vi "Get Item BG Color.vi"(0 "Tree Reference In":refnum<vi>, 1 "Tag (Current)":string, 5 "error in (no error)":errorcluster, 9 "Column # (0)":i32) -> (14 "Tree Reference Out":refnum<vi>, 15 "Duplicate Tag":string, 19 "error out":errorcluster)   [LabVIEW 2015, in "QuickVIew.lvlib"]
doc: "Gets cell BG colorTLB Prime - Application Template 1.3.0.24\nNorm Kirchner, NI Systems Engineering - NI\nCopyright (c) 2014, NI"
uses:
  QuickVIew.lvlib
panel:
  out "Cell BG Color":u32(colorbox)
  # "VI INPUTS"
  # "VI OUTPUTS"
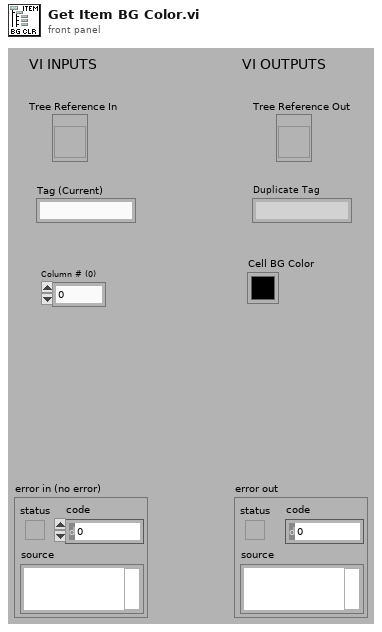
[diagram p1: front panel]
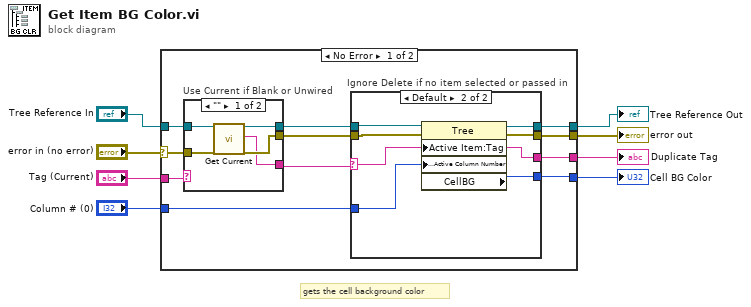
[diagram p0: block diagram]
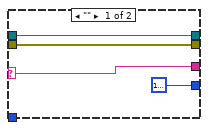
[diagram p2: hidden frame]
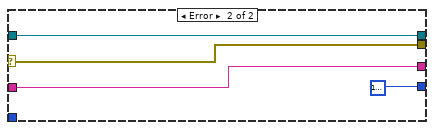
[diagram p4: hidden frame]
diagram:
  # "gets the cell background color"
  n1 = case shown="No Error" "error in (no error)" {
    selector: "error in (no error)" -> [w17 w41]
    tunnel: "Tree Reference In" -> [w19 w42]
    tunnel: [w16 w42] -> w7
    tunnel: [w15 w41] -> w6
    tunnel: "Tag (Current)" -> [w18 w40]
    tunnel: "Column # (0)" -> [w11 _]
    tunnel: [w10 w40] -> w2
    tunnel: [w9 u32 16777226 ("Cell BG Color")] -> w1
    frame No Error {
      n2 = case "Use Current if Blank or Unwired" shown="\"\"" w18 {
        selector: w18 -> [_ w36]
        tunnel: [w34 w38] -> w14
        tunnel: w19 -> [w35 w38]
        tunnel: [w33 w37] -> w13
        tunnel: w17 -> [w32 w37]
        tunnel: [w31 w36] -> w12
        frame "" {
          n3 = call "Get Current.vi"("Tree Reference In"=w35, "error in (no error)"=w32) -> ("Tree Reference Out"=w34:refnum<vi>, "Current Tag"=w31:string, "error out"=w33:errorcluster)  [unwired: 14 in, 1 out]
        }
        frame Default {
        }
      }
      n4 = case "Ignore Delete if no item selected or passed in" shown="Default" w12 {
        selector: w12 -> [w21 w25]
        tunnel: [w23 w27] -> w16
        tunnel: [w22 w26] -> w15
        tunnel: w14 -> [w23 w30]
        tunnel: w13 -> [w22 w29]
        tunnel: w11 -> [_ w28]
        tunnel: [w21 w25] -> w10
        tunnel: [u32 16777226 ("Cell BG Color") w24] -> w9
        frame "" {
        }
        frame Default {
          n5 = property class="Tree"(reference=w30, error in=w29, "Active Item:Tag"=w25, "Active Cell:Active Column Number"=w28) -> (reference out=w27:refnum<vi>, error out=w26:errorcluster, "CellBG"=w24:u32)
        }
      }
    }
    frame Error {
    }
  }
  "Tree Reference Out" <- w7
  "error out" <- w6
  "Duplicate Tag" <- w2
  "Cell BG Color" <- w1
